vi "SVXMPL_Set Display Bounds.vi"(8 "error in (no error)":errorcluster) -> (0 "error out":errorcluster, 2 "display bounds":T1)   [LabVIEW 2017]
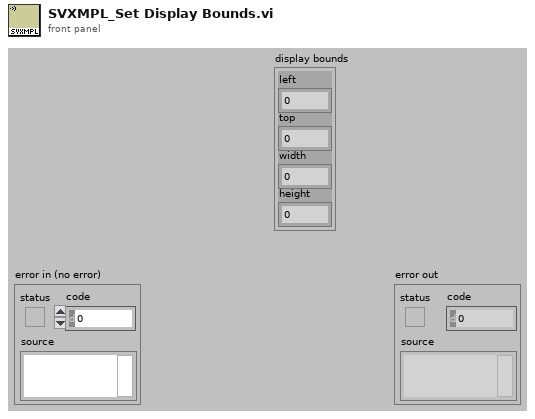
[diagram p1: front panel]
types:
  T1 = cluster{"left":i16, "top":i16, "width":i16, "height":i16}
  T2 = typedef "LVRectTypeDef.ctl" = cluster{"Left":i16, "Top":i16, "Right":i16, "Bottom":i16}
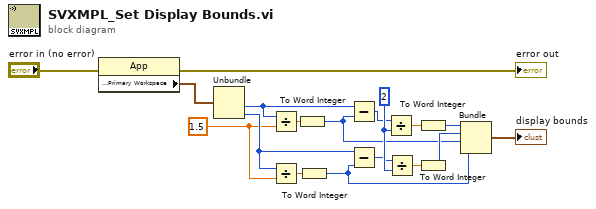
[diagram p0: block diagram]
diagram:
  w5 = 1.5
  w15 = i16 2 ("y")
  n1 = property class="App"(error in="error in (no error)") -> (error out=→"error out":errorcluster, "Display:Primary Workspace"=w3:T2)  [unwired: 1 in, 1 out]
  n2 = Unbundle(w3) -> ("Right"=w4:i16, "Bottom"=w6:i16)  [unwired: 2 out]
  n3 = Divide(x=w4, y=w5) -> (x/y=w7:dbl)
  n4 = Divide(x=w6, y=w5) -> (x/y=w8:dbl)
  n5 = To Word Integer(number=w7) -> (16bit integer=w9:i16)
  n6 = To Word Integer(number=w8) -> (16bit integer=w10:i16)
  n7 = Subtract(x=w4, y=w9) -> (x-y=w11:i16)
  n8 = Subtract(x=w6, y=w10) -> (x-y=w14:i16)
  n9 = Divide(x=w11, y=w15) -> (x/y=w12:dbl)
  n10 = Divide(x=w14, y=w15) -> (x/y=w16:dbl)
  n11 = To Word Integer(number=w12) -> (16bit integer=w13:i16)
  n12 = To Word Integer(number=w16) -> (16bit integer=w17:i16)
  n13 = Bundle(w13, w17, w9, w10) -> (→"display bounds":cluster{i16, i16, i16, i16})  [unwired: 1 in]
